vi "Hardware Out - NI 9754-1 (ESTTL).vi"(0 "FPGA Ref":T3, 11 "RT Data in":T1={"Refs"={"FPGA 1"=refnum, "FPGA 2"=refnum}, "EPT"={"MaxCAD"=0.0, "EPT Sim Enabled"=FALSE, "EPTxData"={"Sync"=FALSE, "CurrentCAD"=0.0, "Speed [RPM]"=0.0, "Config"=FALSE, "Rcvg Primary"=FALSE, "Stall"=FALSE, "Overflow"=FALSE, "Ratio Error"=FALSE, "Pattern Error"=FALSE, "Aux Warning"=FALSE, "Watchdog Error"=FALSE}}, "Raw Inputs"={"NI9752s"=[], "NI9757s"=[], "NI9411s"=[], "NI9220s"=[], "VRHalls"=[]}, "Control Inputs"={"Engine Speed [RPM]"=0.0, "Engine Status"=enum."STALLED", "Load Control \nMode"=enum."High-Idle Governor", "dt(s)"=0.0, "Number of Cylinders"=0, "Engine Displacement [cc]"=0.0, "StoichAFR"=0.0, "Q.LHV Fuel [kJ/kg]"=0.0, "BattV PSU [V]"=0.0, "12V PSU [V]"=0.0, "5V PSU [V]"=0.0, "Pedal Position [%]"=0.0, "Oil Pressure [kPa]"=0.0, "Oil Temp [C]"=0.0, "Oil Level [%]"=0.0, "Engine Coolant Temp (ECT) [C]"=0.0, "Engine Coolant Pressure [kPa]"=0.0, "Rail Pressure [bar]"=0.0, "Fuel Pressure [kPa]"=0.0, "Fuel Temp [C]"=0.0, "Vacuum Pressure [kPa]"=0.0, "Throttle Position [%]"=0.0, "Cam1 Advance [CAD]"=0.0, "Cam2 Advance [CAD]"=0.0, "Cam3 Advance [CAD]"=0.0, "Cam4 Advance [CAD]"=0.0, "CA50 Control Output [CAD]"=[], "CA50 Control Output Valid"=[], "Intake Air Temp (IAT) [C]"=0.0, "Barometric Air Pressure [kPa]"=0.0, "Intake Air Rel. Humidity [%]"=0.0, "Mass Air Flow (MAF) [kg/hr]"=0.0, "Turbo Inlet Air Pressure [kPa]"=0.0, "Turbo Inlet Air Temp [C]"=0.0, "Turbo Outlet Air Pressure [kPa]"=0.0, "Turbo Outlet Air Temp [C]"=0.0, "CAC Outlet Pressure [kPa]"=0.0, "CAC Outlet Temp [C]"=0.0, "Intake Manifold Pressure (MAP) [kPa]"=0.0, "Intake Manifold Temp (MAT) [C]"=0.0, "Exhaust Manifold Pressure [kPa]"=0.0, "Exhaust Manifold Temp [C]"=0.0, "HighP EGR Cooler Outlet Pressure [kPa]"=0.0, "HighP EGR Cooler Outlet Temp [C]"=0.0, "HighP EGR Differential Pressure [kPa]"=0.0, "HighP EGR Valve Position [%]"=0.0, "Turbo Outlet Exhaust Pressure [kPa]"=0.0, "Turbo Outlet Exhaust Temp [C]"=0.0, "VGT Position 1 [%]"=0.0, "VGT Position 2 [%]"=0.0, "Turbo Speed 1 [RPM]"=0.0, "Turbo Speed 2 [RPM]"=0.0, "LowP EGR Differential Pressure [kPa]"=0.0, "LowP EGR Valve Position [%]"=0.0, "UEGO1Lambda"=0.0, "UEGO1_Hot"=FALSE, "UEGO2Lambda"=0.0, "UEGO2_Hot"=FALSE, "Knock Intensity"=[], "Knock"=[]}, "Control Outputs"={"Pedal Desired [%]"=0.0, "MEP Desired [bar]"=0.0, "Fuel Desired [mg/cyc]"=0.0, "Intake MAP Desired [kPa]"=0.0, "Cam1 Advance Setpoint [CAD]"=0.0, "Cam2 Advance Setpoint [CAD]"=0.0, "HighP EGR Position Setpoint [%Open]"=0.0, "LowP EGR Position Setpoint [%Open]"=0.0, "Rail Pressure Setpoint [bar]"=0.0, "Wastegate1 Position Setpoint [%Open]"=0.0, "Wastegate2 Position Setpoint [%Open]"=0.0, "VGT1 Position Setpoint [%Open]"=0.0, "VGT2 Position Setpoint [%Open]"=0.0, "Throttle1 Position Setpoint [%Open]"=0.0, "Throttle2 Position Setpoint [%Open]"=0.0, "TurboBPV Position Setpoint [%Open]"=0.0, "Spark Dwells [msec]"=[], "Spark Timings [DBTDC]"=[], "PFI Quantities [mg/inj]"=[], "PFI Timings [DBTDC]"=[], "DI Quantities [mg/inj]"=[], "DI Timings [DBTDC]"=[]}, "Raw Outputs"={"9751-1"={"DI1"={"Window_Start (DBTDC)"=0.0, "Window_End (DBTDC)"=0.0, "Enable_Inj1"=FALSE, "Duration_Inj1 (msec)"=0.0, "Timing_Inj1 (DBTDC)"=0.0, "Enable_Inj2"=FALSE, "Duration_Inj2 (msec)"=0.0, "Timing_Inj2 (DBTDC)"=0.0, "Enable_Inj3"=FALSE, "Duration_Inj3 (msec)"=0.0, "Timing_Inj3 (DBTDC)"=0.0, "Enable_Inj4"=FALSE, "Duration_Inj4 (msec)"=0.0, "Timing_Inj4 (DBTDC)"=0.0, "Enable_Inj5"=FALSE, "Duration_Inj5 (msec)"=0.0, "Timing_Inj5 (DBTDC)"=0.0}, "DI2"={"Window_Start (DBTDC)"=0.0, "Window_End (DBTDC)"=0.0, "Enable_Inj1"=FALSE, "Duration_Inj1 (msec)"=0.0, "Timing_Inj1 (DBTDC)"=0.0, "Enable_Inj2"=FALSE, "Duration_Inj2 (msec)"=0.0, "Timing_Inj2 (DBTDC)"=0.0, "Enable_Inj3"=FALSE, "Duration_Inj3 (msec)"=0.0, "Timing_Inj3 (DBTDC)"=0.0, "Enable_Inj4"=FALSE, "Duration_Inj4 (msec)"=0.0, "Timing_Inj4 (DBTDC)"=0.0, "Enable_Inj5"=FALSE, "Duration_Inj5 (msec)"=0.0, "Timing_Inj5 (DBTDC)"=0.0}, "DI3"={"Window_Start (DBTDC)"=0.0, "Window_End (DBTDC)"=0.0, "Enable_Inj1"=FALSE, "Duration_Inj1 (msec)"=0.0, "Timing_Inj1 (DBTDC)"=0.0, "Enable_Inj2"=FALSE, "Duration_Inj2 (msec)"=0.0, "Timing_Inj2 (DBTDC)"=0.0, "Enable_Inj3"=FALSE, "Duration_Inj3 (msec)"=0.0, "Timing_Inj3 (DBTDC)"=0.0, "Enable_Inj4"=FALSE, "Duration_Inj4 (msec)"=0.0, "Timing_Inj4 (DBTDC)"=0.0, "Enable_Inj5"=FALSE, "Duration_Inj5 (msec)"=0.0, "Timing_Inj5 (DBTDC)"=0.0}}, "9751-2"={"DI1"={"Window_Start (DBTDC)"=0.0, "Window_End (DBTDC)"=0.0, "Enable_Inj1"=FALSE, "Duration_Inj1 (msec)"=0.0, "Timing_Inj1 (DBTDC)"=0.0, "Enable_Inj2"=FALSE, "Duration_Inj2 (msec)"=0.0, "Timing_Inj2 (DBTDC)"=0.0, "Enable_Inj3"=FALSE, "Duration_Inj3 (msec)"=0.0, "Timing_Inj3 (DBTDC)"=0.0, "Enable_Inj4"=FALSE, "Duration_Inj4 (msec)"=0.0, "Timing_Inj4 (DBTDC)"=0.0, "Enable_Inj5"=FALSE, "Duration_Inj5 (msec)"=0.0, "Timing_Inj5 (DBTDC)"=0.0}, "DI2"={"Window_Start (DBTDC)"=0.0, "Window_End (DBTDC)"=0.0, "Enable_Inj1"=FALSE, "Duration_Inj1 (msec)"=0.0, "Timing_Inj1 (DBTDC)"=0.0, "Enable_Inj2"=FALSE, "Duration_Inj2 (msec)"=0.0, "Timing_Inj2 (DBTDC)"=0.0, "Enable_Inj3"=FALSE, "Duration_Inj3 (msec)"=0.0, "Timing_Inj3 (DBTDC)"=0.0, "Enable_Inj4"=FALSE, "Duration_Inj4 (msec)"=0.0, "Timing_Inj4 (DBTDC)"=0.0, "Enable_Inj5"=FALSE, "Duration_Inj5 (msec)"=0.0, "Timing_Inj5 (DBTDC)"=0.0}, "DI3"={"Window_Start (DBTDC)"=0.0, "Window_End (DBTDC)"=0.0, "Enable_Inj1"=FALSE, "Duration_Inj1 (msec)"=0.0, "Timing_Inj1 (DBTDC)"=0.0, "Enable_Inj2"=FALSE, "Duration_Inj2 (msec)"=0.0, "Timing_Inj2 (DBTDC)"=0.0, "Enable_Inj3"=FALSE, "Duration_Inj3 (msec)"=0.0, "Timing_Inj3 (DBTDC)"=0.0, "Enable_Inj4"=FALSE, "Duration_Inj4 (msec)"=0.0, "Timing_Inj4 (DBTDC)"=0.0, "Enable_Inj5"=FALSE, "Duration_Inj5 (msec)"=0.0, "Timing_Inj5 (DBTDC)"=0.0}}, "9751-3"={"DI1"={"Window_Start (DBTDC)"=0.0, "Window_End (DBTDC)"=0.0, "Enable_Inj1"=FALSE, "Duration_Inj1 (msec)"=0.0, "Timing_Inj1 (DBTDC)"=0.0, "Enable_Inj2"=FALSE, "Duration_Inj2 (msec)"=0.0, "Timing_Inj2 (DBTDC)"=0.0, "Enable_Inj3"=FALSE, "Duration_Inj3 (msec)"=0.0, "Timing_Inj3 (DBTDC)"=0.0, "Enable_Inj4"=FALSE, "Duration_Inj4 (msec)"=0.0, "Timing_Inj4 (DBTDC)"=0.0, "Enable_Inj5"=FALSE, "Duration_Inj5 (msec)"=0.0, "Timing_Inj5 (DBTDC)"=0.0}, "DI2"={"Window_Start (DBTDC)"=0.0, "Window_End (DBTDC)"=0.0, "Enable_Inj1"=FALSE, "Duration_Inj1 (msec)"=0.0, "Timing_Inj1 (DBTDC)"=0.0, "Enable_Inj2"=FALSE, "Duration_Inj2 (msec)"=0.0, "Timing_Inj2 (DBTDC)"=0.0, "Enable_Inj3"=FALSE, "Duration_Inj3 (msec)"=0.0, "Timing_Inj3 (DBTDC)"=0.0, "Enable_Inj4"=FALSE, "Duration_Inj4 (msec)"=0.0, "Timing_Inj4 (DBTDC)"=0.0, "Enable_Inj5"=FALSE, "Duration_Inj5 (msec)"=0.0, "Timing_Inj5 (DBTDC)"=0.0}, "DI3"={"Window_Start (DBTDC)"=0.0, "Window_End (DBTDC)"=0.0, "Enable_Inj1"=FALSE, "Duration_Inj1 (msec)"=0.0, "Timing_Inj1 (DBTDC)"=0.0, "Enable_Inj2"=FALSE, "Duration_Inj2 (msec)"=0.0, "Timing_Inj2 (DBTDC)"=0.0, "Enable_Inj3"=FALSE, "Duration_Inj3 (msec)"=0.0, "Timing_Inj3 (DBTDC)"=0.0, "Enable_Inj4"=FALSE, "Duration_Inj4 (msec)"=0.0, "Timing_Inj4 (DBTDC)"=0.0, "Enable_Inj5"=FALSE, "Duration_Inj5 (msec)"=0.0, "Timing_Inj5 (DBTDC)"=0.0}}, "9751-4"={"DI1"={"Window_Start (DBTDC)"=0.0, "Window_End (DBTDC)"=0.0, "Enable_Inj1"=FALSE, "Duration_Inj1 (msec)"=0.0, "Timing_Inj1 (DBTDC)"=0.0, "Enable_Inj2"=FALSE, "Duration_Inj2 (msec)"=0.0, "Timing_Inj2 (DBTDC)"=0.0, "Enable_Inj3"=FALSE, "Duration_Inj3 (msec)"=0.0, "Timing_Inj3 (DBTDC)"=0.0, "Enable_Inj4"=FALSE, "Duration_Inj4 (msec)"=0.0, "Timing_Inj4 (DBTDC)"=0.0, "Enable_Inj5"=FALSE, "Duration_Inj5 (msec)"=0.0, "Timing_Inj5 (DBTDC)"=0.0}, "DI2"={"Window_Start (DBTDC)"=0.0, "Window_End (DBTDC)"=0.0, "Enable_Inj1"=FALSE, "Duration_Inj1 (msec)"=0.0, "Timing_Inj1 (DBTDC)"=0.0, "Enable_Inj2"=FALSE, "Duration_Inj2 (msec)"=0.0, "Timing_Inj2 (DBTDC)"=0.0, "Enable_Inj3"=FALSE, "Duration_Inj3 (msec)"=0.0, "Timing_Inj3 (DBTDC)"=0.0, "Enable_Inj4"=FALSE, "Duration_Inj4 (msec)"=0.0, "Timing_Inj4 (DBTDC)"=0.0, "Enable_Inj5"=FALSE, "Duration_Inj5 (msec)"=0.0, "Timing_Inj5 (DBTDC)"=0.0}, "DI3"={"Window_Start (DBTDC)"=0.0, "Window_End (DBTDC)"=0.0, "Enable_Inj1"=FALSE, "Duration_Inj1 (msec)"=0.0, "Timing_Inj1 (DBTDC)"=0.0, "Enable_Inj2"=FALSE, "Duration_Inj2 (msec)"=0.0, "Timing_Inj2 (DBTDC)"=0.0, "Enable_Inj3"=FALSE, "Duration_Inj3 (msec)"=0.0, "Timing_Inj3 (DBTDC)"=0.0, "Enable_Inj4"=FALSE, "Duration_Inj4 (msec)"=0.0, "Timing_Inj4 (DBTDC)"=0.0, "Enable_Inj5"=FALSE, "Duration_Inj5 (msec)"=0.0, "Timing_Inj5 (DBTDC)"=0.0}}, "9754-1"={"ESTTL 1"={"Timing (DBTDC)"=0.0, "Dwell (ms)"=0.0}, "ESTTL 2"={"Timing (DBTDC)"=0.0, "Dwell (ms)"=0.0}, "ESTTL 3"={"Timing (DBTDC)"=0.0, "Dwell (ms)"=0.0}, "ESTTL 4"={"Timing (DBTDC)"=0.0, "Dwell (ms)"=0.0}, "ESTTL 5"={"Timing (DBTDC)"=0.0, "Dwell (ms)"=0.0}, "ESTTL 6"={"Timing (DBTDC)"=0.0, "Dwell (ms)"=0.0}, "ESTTL 7"={"Timing (DBTDC)"=0.0, "Dwell (ms)"=0.0}, "ESTTL 8"={"Timing (DBTDC)"=0.0, "Dwell (ms)"=0.0}}, "9754-2"={"ESTTL 1"={"Timing (DBTDC)"=0.0, "Dwell (ms)"=0.0}, "ESTTL 2"={"Timing (DBTDC)"=0.0, "Dwell (ms)"=0.0}, "ESTTL 3"={"Timing (DBTDC)"=0.0, "Dwell (ms)"=0.0}, "ESTTL 4"={"Timing (DBTDC)"=0.0, "Dwell (ms)"=0.0}, "ESTTL 5"={"Timing (DBTDC)"=0.0, "Dwell (ms)"=0.0}, "ESTTL 6"={"Timing (DBTDC)"=0.0, "Dwell (ms)"=0.0}, "ESTTL 7"={"Timing (DBTDC)"=0.0, "Dwell (ms)"=0.0}, "ESTTL 8"={"Timing (DBTDC)"=0.0, "Dwell (ms)"=0.0}}, "9758-1"={"LS 1"={"Enable"=FALSE, "Freq [Hz]"=0.0, "DutyCyc [%]"=0.0}, "LS 2"={"Enable"=FALSE, "Freq [Hz]"=0.0, "DutyCyc [%]"=0.0}, "LS 3"={"Enable"=FALSE, "Freq [Hz]"=0.0, "DutyCyc [%]"=0.0}, "LS 4"={"Enable"=FALSE, "Freq [Hz]"=0.0, "DutyCyc [%]"=0.0}, "PFI 1"={"Position Mode"=FALSE, "Timing (DBTDC)"=0.0, "Pulse Width (ms)"=0.0}, "PFI 2"={"Position Mode"=FALSE, "Timing (DBTDC)"=0.0, "Pulse Width (ms)"=0.0}, "PFI 3"={"Position Mode"=FALSE, "Timing (DBTDC)"=0.0, "Pulse Width (ms)"=0.0}, "PFI 4"={"Position Mode"=FALSE, "Timing (DBTDC)"=0.0, "Pulse Width (ms)"=0.0}}, "9758-2"={"LS 1"={"Enable"=FALSE, "Freq [Hz]"=0.0, "DutyCyc [%]"=0.0}, "LS 2"={"Enable"=FALSE, "Freq [Hz]"=0.0, "DutyCyc [%]"=0.0}, "LS 3"={"Enable"=FALSE, "Freq [Hz]"=0.0, "DutyCyc [%]"=0.0}, "LS 4"={"Enable"=FALSE, "Freq [Hz]"=0.0, "DutyCyc [%]"=0.0}, "PFI 1"={"Position Mode"=FALSE, "Timing (DBTDC)"=0.0, "Pulse Width (ms)"=0.0}, "PFI 2"={"Position Mode"=FALSE, "Timing (DBTDC)"=0.0, "Pulse Width (ms)"=0.0}, "PFI 3"={"Position Mode"=FALSE, "Timing (DBTDC)"=0.0, "Pulse Width (ms)"=0.0}, "PFI 4"={"Position Mode"=FALSE, "Timing (DBTDC)"=0.0, "Pulse Width (ms)"=0.0}}, "9759-1"={"THR1-1 DC [%]"=0.0, "THR1-1 Setpoint [% Open]"=0.0, "THR1-2 DC [%]"=0.0, "THR1-2 Setpoint [% Open]"=0.0}}} {"Control Inputs"."Knock Intensity" format="%.2f"; "Control Inputs"."CA50 Control Output [CAD]" format="%.2f"; "Control Inputs"."Exhaust Manifold Temp [C]" format="%#_6f"; "Control Inputs"."UEGO2Lambda" format="%.2f"; "Control Inputs"."Intake Manifold Temp (MAT) [C]" format="%#_6f"; "Control Inputs"."UEGO1Lambda" format="%.2f"}) -> ()   [LabVIEW 2015, in "ECS-RT.lvlib"]
uses:
  ECS-RT.lvlib
  Typedefs/FPGA Refs/Generic FPGA Ref.ctl
  Typedefs/RT Data.ctl
  Typedefs/FPGA Refs/FPGA Refs.ctl
  Typedefs/EPT/EPT Cluster.ctl
  <vilib>/Powertrain Controls/Device Drivers/Engine Position Tracking/EPTx/RevA/RT/Controls/EPTxData.ctl
  Typedefs/Raw Inputs/Raw Inputs.ctl
  Typedefs/Raw Inputs/NI9752.ctl
  Typedefs/Raw Inputs/PPWData.ctl
  Typedefs/Raw Inputs/NI9757.ctl
  Typedefs/Raw Inputs/NI9411.ctl
  Typedefs/Raw Inputs/NI9220.ctl
  Typedefs/Raw Inputs/VRHall.ctl
  Typedefs/Control Inputs/Control Inputs.ctl
  Typedefs/EPT/Engine Status.ctl
  Typedefs/MISC/Load Control Mode.ctl
  Typedefs/Control Outputs/Control Outputs.ctl
  Typedefs/Control Outputs/Injection Quantity.ctl
  Typedefs/Control Outputs/Injection Timing.ctl
  Typedefs/Raw Outputs/Raw Outputs.ctl
  Typedefs/Raw Outputs/NI9751.ctl
  Typedefs/Raw Outputs/DI.ctl
  Typedefs/Raw Outputs/NI9754.ctl
  Typedefs/Raw Outputs/ESTTL.ctl
  Typedefs/Raw Outputs/NI9758.ctl
  Typedefs/Raw Outputs/LS.ctl
  Typedefs/Raw Outputs/PFI.ctl
  Typedefs/Raw Outputs/NI9759.ctl
  <vilib>/Utility/error.llb/Error Cluster From Error Code.vi
  <vilib>/rvi/errors/niLvFpgaAdjustHostInterfaceError.vi
  Globals/TDC Globals.vi
  <vilib>/rvi/interface/nirviReadWriteControl/nirviReadWriteControl.xnode
  <vilib>/rvi/interface/Simulation/niFpgaSimulationCallBeginRW.vi
  NiFpgaLv.dll
  <vilib>/Powertrain Controls/Device Drivers/Engine Position Tracking/EPTx/RevA/RT/EPTx - RevA - RT.lvlib
  ECS-Shared.lvlib
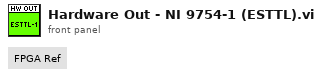
[diagram p1: front panel]
types:
  T1 = typedef "ECS-Shared.lvlib/RT Data.ctl" = cluster{"Refs":T2, "EPT":T4, "Raw Inputs":T6, "Control Inputs":T13, "Control Outputs":T16, "Raw Outputs":T19}
  T2 = typedef "ECS-Shared.lvlib/FPGA Refs.ctl" = cluster{"FPGA 1":T3, "FPGA 2":T3}
  T3 = typedef "ECS-Shared.lvlib/Generic FPGA Ref.ctl" = refnum<k20>
  T4 = typedef "ECS-Shared.lvlib/EPT Cluster.ctl" = cluster{"MaxCAD":sgl, "EPT Sim Enabled":bool, "EPTxData":T5}
  T5 = typedef "EPTx - RevA - RT.lvlib/EPTxData.ctl" = cluster{"Sync":bool, "CurrentCAD":sgl, "Speed [RPM]":sgl, "Config":bool, "Rcvg Primary":bool, "Stall":bool, "Overflow":bool, "Ratio Error":bool, "Pattern Error":bool, "Aux Warning":bool, "Watchdog Error":bool}
  T6 = typedef "ECS-Shared.lvlib/Raw Inputs.ctl" = cluster{"NI9752s":T7[], "NI9757s":T9[], "NI9411s":T10[], "NI9220s":T11[], "VRHalls":T12[]}
  T7 = typedef "ECS-Shared.lvlib/NI9752.ctl" = cluster{"Voltage [V]":sgl[], "Resistance [Ohm]":sgl[], "PPWData VR1":T8, "PPWData VR2":T8, "PPWData Hall1":T8, "PPWData Hall2":T8}
  T8 = typedef "ECS-Shared.lvlib/PPWData.ctl" = cluster{"Period":u32, "PulseWidth":u32, "Stopped":bool}
  T9 = typedef "ECS-Shared.lvlib/NI9757.ctl" = cluster{"UEGO1":cluster{"Lambda":sgl, "Phi":sgl, "AF_Ratio":sgl, "Ip":sgl, "Temp":sgl, "Hot":bool}, "UEGO2":cluster{"Lambda":sgl, "Phi":sgl, "AF_Ratio":sgl, "Ip":sgl, "Temp":sgl, "Hot":bool}, "EGO1":cluster{"Status":enum16{"COLD SENSOR", "FOULED SENSOR", "RICH", "LEAN"}, "SensorV":sgl}, "EGO2":cluster{"Status":enum16{"COLD SENSOR", "FOULED SENSOR", "RICH", "LEAN"}, "SensorV":sgl}, "EGO3":cluster{"Status":enum16{"COLD SENSOR", "FOULED SENSOR", "RICH", "LEAN"}, "SensorV":sgl}, "EGO4":cluster{"Status":enum16{"COLD SENSOR", "FOULED SENSOR", "RICH", "LEAN"}, "SensorV":sgl}}
  T10 = typedef "ECS-Shared.lvlib/NI9411.ctl" = cluster{"PPWData 0":T8, "PPWData 1":T8, "PPWData 2":T8, "PPWData 3":T8, "PPWData 4":T8, "PPWData 5":T8}
  T11 = typedef "ECS-Shared.lvlib/NI9220.ctl" = cluster{"AI 0":sgl, "AI 1":sgl, "AI 2":sgl, "AI 3":sgl, "AI 4":sgl, "AI 5":sgl, "AI 6":sgl, "AI 7":sgl, "AI 8":sgl, "AI 9":sgl, "AI 10":sgl, "AI 11":sgl, "AI 12":sgl, "AI 13":sgl, "AI 14":sgl, "AI 15":sgl}
  T12 = typedef "ECS-Shared.lvlib/VRHall.ctl" = cluster{"PPWData 0":T8, "PPWData 1":T8, "PPWData 2":T8, "PPWData 3":T8, "PPWData 4":T8, "PPWData 5":T8}
  T13 = typedef "ECS-Shared.lvlib/Control Inputs.ctl" = cluster{"Engine Speed [RPM]":sgl, "Engine Status":T14, "Load Control \nMode":T15, "dt(s)":sgl, "Number of Cylinders":u8, "Engine Displacement [cc]":sgl, "StoichAFR":sgl, "Q.LHV Fuel [kJ/kg]":sgl, "BattV PSU [V]":sgl, "12V PSU [V]":sgl, "5V PSU [V]":sgl, "Pedal Position [%]":sgl, "Oil Pressure [kPa]":sgl, "Oil Temp [C]":sgl, "Oil Level [%]":sgl, "Engine Coolant Temp (ECT) [C]":sgl, "Engine Coolant Pressure [kPa]":sgl, "Rail Pressure [bar]":sgl, "Fuel Pressure [kPa]":sgl, "Fuel Temp [C]":sgl, "Vacuum Pressure [kPa]":sgl, "Throttle Position [%]":sgl, "Cam1 Advance [CAD]":sgl, "Cam2 Advance [CAD]":sgl, "Cam3 Advance [CAD]":sgl, "Cam4 Advance [CAD]":sgl, "CA50 Control Output [CAD]":sgl[], "CA50 Control Output Valid":bool[], "Intake Air Temp (IAT) [C]":sgl, "Barometric Air Pressure [kPa]":sgl, "Intake Air Rel. Humidity [%]":sgl, "Mass Air Flow (MAF) [kg/hr]":sgl, "Turbo Inlet Air Pressure [kPa]":sgl, "Turbo Inlet Air Temp [C]":sgl, "Turbo Outlet Air Pressure [kPa]":sgl, "Turbo Outlet Air Temp [C]":sgl, "CAC Outlet Pressure [kPa]":sgl, "CAC Outlet Temp [C]":sgl, "Intake Manifold Pressure (MAP) [kPa]":sgl, "Intake Manifold Temp (MAT) [C]":sgl, "Exhaust Manifold Pressure [kPa]":sgl, "Exhaust Manifold Temp [C]":sgl, "HighP EGR Cooler Outlet Pressure [kPa]":sgl, "HighP EGR Cooler Outlet Temp [C]":sgl, "HighP EGR Differential Pressure [kPa]":sgl, "HighP EGR Valve Position [%]":sgl, "Turbo Outlet Exhaust Pressure [kPa]":sgl, "Turbo Outlet Exhaust Temp [C]":sgl, "VGT Position 1 [%]":sgl, "VGT Position 2 [%]":sgl, "Turbo Speed 1 [RPM]":sgl, "Turbo Speed 2 [RPM]":sgl, "LowP EGR Differential Pressure [kPa]":sgl, "LowP EGR Valve Position [%]":sgl, "UEGO1Lambda":sgl, "UEGO1_Hot":bool, "UEGO2Lambda":sgl, "UEGO2_Hot":bool, "Knock Intensity":sgl[], "Knock":bool[]}
  T14 = typedef "ECS-Shared.lvlib/Engine Status.ctl" = enum16{"OFF", "STALLED", "CRANKING", "RUNNING", "ACCEL", "DECEL", "SAFE"}
  T15 = typedef "ECS-Shared.lvlib/Load Control Mode.ctl" = enum16{"No Governor", "Low-Idle Governor", "High-Idle Governor"}
  T16 = typedef "ECS-Shared.lvlib/Control Outputs.ctl" = cluster{"Pedal Desired [%]":sgl, "MEP Desired [bar]":sgl, "Fuel Desired [mg/cyc]":sgl, "Intake MAP Desired [kPa]":sgl, "Cam1 Advance Setpoint [CAD]":sgl, "Cam2 Advance Setpoint [CAD]":sgl, "HighP EGR Position Setpoint [%Open]":sgl, "LowP EGR Position Setpoint [%Open]":sgl, "Rail Pressure Setpoint [bar]":sgl, "Wastegate1 Position Setpoint [%Open]":sgl, "Wastegate2 Position Setpoint [%Open]":sgl, "VGT1 Position Setpoint [%Open]":sgl, "VGT2 Position Setpoint [%Open]":sgl, "Throttle1 Position Setpoint [%Open]":sgl, "Throttle2 Position Setpoint [%Open]":sgl, "TurboBPV Position Setpoint [%Open]":sgl, "Spark Dwells [msec]":sgl[], "Spark Timings [DBTDC]":sgl[], "PFI Quantities [mg/inj]":sgl[], "PFI Timings [DBTDC]":sgl[], "DI Quantities [mg/inj]":T17[], "DI Timings [DBTDC]":T18[]}
  T17 = typedef "ECS-Shared.lvlib/Injection Quantity.ctl" = cluster{"Pilot1Quantity [mg/inj]":sgl, "Pilot2Quantity [mg/inj]":sgl, "MainQuantity [mg/inj]":sgl, "Post1Quantity [mg/inj]":sgl, "Post2Quantity [mg/inj]":sgl}
  T18 = typedef "ECS-Shared.lvlib/Injection Timing.ctl" = cluster{"Pilot1SOI [DBTDC]":sgl, "Pilot2SOI [DBTDC]":sgl, "MainSOI [DBTDC]":sgl, "Post1SOI [DBTDC]":sgl, "Post2SOI [DBTDC]":sgl}
  T19 = typedef "ECS-Shared.lvlib/Raw Outputs.ctl" = cluster{"9751-1":T20, "9751-2":T20, "9751-3":T20, "9751-4":T20, "9754-1":T22, "9754-2":T22, "9758-1":T24, "9758-2":T24, "9759-1":T27}
  T20 = typedef "ECS-Shared.lvlib/NI9751.ctl" = cluster{"DI1":T21, "DI2":T21, "DI3":T21}
  T21 = typedef "ECS-Shared.lvlib/DI.ctl" = cluster{"Window_Start (DBTDC)":sgl, "Window_End (DBTDC)":sgl, "Enable_Inj1":bool, "Duration_Inj1 (msec)":sgl, "Timing_Inj1 (DBTDC)":sgl, "Enable_Inj2":bool, "Duration_Inj2 (msec)":sgl, "Timing_Inj2 (DBTDC)":sgl, "Enable_Inj3":bool, "Duration_Inj3 (msec)":sgl, "Timing_Inj3 (DBTDC)":sgl, "Enable_Inj4":bool, "Duration_Inj4 (msec)":sgl, "Timing_Inj4 (DBTDC)":sgl, "Enable_Inj5":bool, "Duration_Inj5 (msec)":sgl, "Timing_Inj5 (DBTDC)":sgl}
  T22 = typedef "ECS-Shared.lvlib/NI9754.ctl" = cluster{"ESTTL 1":T23, "ESTTL 2":T23, "ESTTL 3":T23, "ESTTL 4":T23, "ESTTL 5":T23, "ESTTL 6":T23, "ESTTL 7":T23, "ESTTL 8":T23}
  T23 = typedef "ECS-Shared.lvlib/ESTTL.ctl" = cluster{"Timing (DBTDC)":sgl, "Dwell (ms)":sgl}
  T24 = typedef "ECS-Shared.lvlib/NI9758.ctl" = cluster{"LS 1":T25, "LS 2":T25, "LS 3":T25, "LS 4":T25, "PFI 1":T26, "PFI 2":T26, "PFI 3":T26, "PFI 4":T26}
  T25 = typedef "ECS-Shared.lvlib/LS.ctl" = cluster{"Enable":bool, "Freq [Hz]":sgl, "DutyCyc [%]":sgl}
  T26 = typedef "ECS-Shared.lvlib/PFI.ctl" = cluster{"Position Mode":bool, "Timing (DBTDC)":sgl, "Pulse Width (ms)":sgl}
  T27 = typedef "ECS-Shared.lvlib/NI9759.ctl" = cluster{"THR1-1 DC [%]":sgl, "THR1-1 Setpoint [% Open]":sgl, "THR1-2 DC [%]":sgl, "THR1-2 Setpoint [% Open]":sgl}
  T28 = cluster{"Channel Enable 1":bool, "Window_Start 1 [CAD]":fxp<+,18,11>, "Window_End 1 [CAD]":fxp<+,18,11>, "Dwell 1 [ms]":fxp<+/-,22,9>, "Spark Timing 1 [CAD]":fxp<+,18,11>, "Channel Enable 2":bool, "Window_Start 2 [CAD]":fxp<+,18,11>, "Window_End 2 [CAD]":fxp<+,18,11>, "Dwell 2 [ms]":fxp<+/-,22,9>, "Spark Timing 2 [CAD]":fxp<+,18,11>, "Channel Enable 3":bool, "Window_Start 3 [CAD]":fxp<+,18,11>, "Window_End 3 [CAD]":fxp<+,18,11>, "Dwell 3 [ms]":fxp<+/-,22,9>, "Spark Timing 3 [CAD]":fxp<+,18,11>, "Channel Enable 4":bool, "Window_Start 4 [CAD]":fxp<+,18,11>, "Window_End 4 [CAD]":fxp<+,18,11>, "Dwell 4 [ms]":fxp<+/-,22,9>, "Spark Timing 4 [CAD]":fxp<+,18,11>, "Channel Enable 5":bool, "Window_Start 5 [CAD]":fxp<+,18,11>, "Window_End 5 [CAD]":fxp<+,18,11>, "Dwell 5 [ms]":fxp<+/-,22,9>, "Spark Timing 5 [CAD]":fxp<+,18,11>, "Channel Enable 6":bool, "Window_Start 6 [CAD]":fxp<+,18,11>, "Window_End 6 [CAD]":fxp<+,18,11>, "Dwell 6 [ms]":fxp<+/-,22,9>, "Spark Timing 6 [CAD]":fxp<+,18,11>, "Channel Enable 7":bool, "Window_Start 7 [CAD]":fxp<+,18,11>, "Window_End 7 [CAD]":fxp<+,18,11>, "Dwell 7 [ms]":fxp<+/-,22,9>, "Spark Timing 7 [CAD]":fxp<+,18,11>, "Channel Enable 8":bool, "Window_Start 8 [CAD]":fxp<+,18,11>, "Window_End 8 [CAD]":fxp<+,18,11>, "Dwell 8 [ms]":fxp<+/-,22,9>, "Spark Timing 8 [CAD]":fxp<+,18,11>}
  T29 = cluster{"DurationSeq":u32[], "CmdLevelSeq":bool[], "ContinueSeq":bool[]}
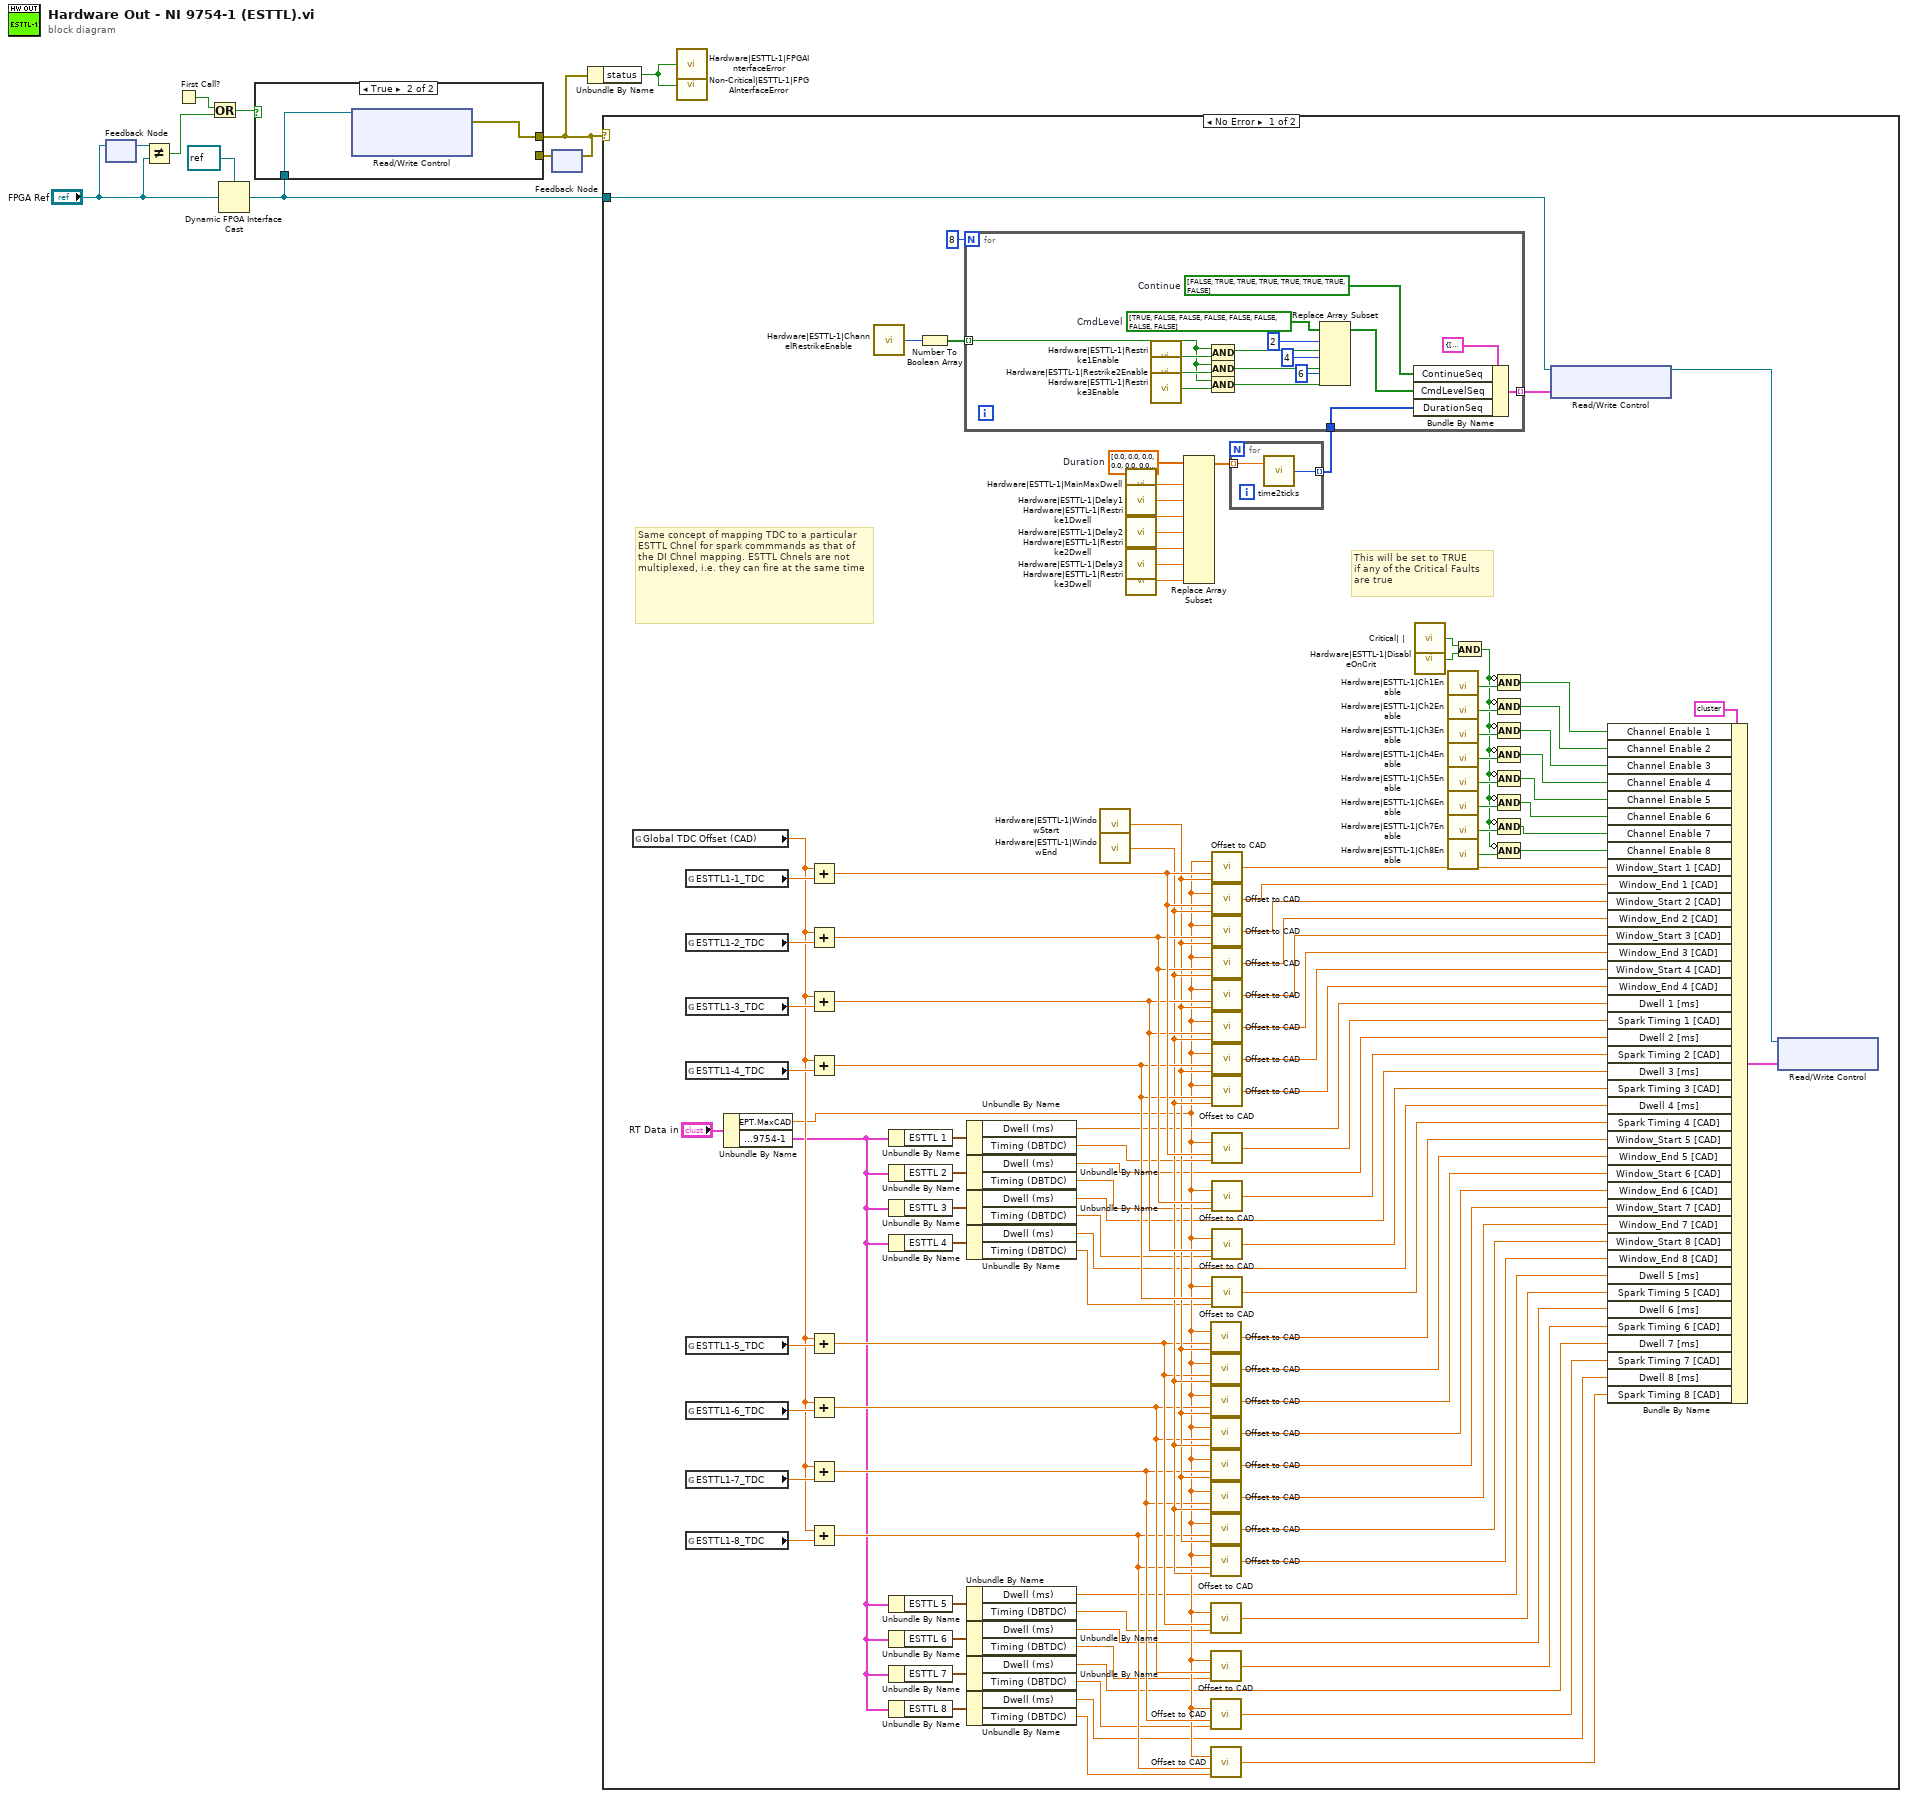
[diagram p0: block diagram]
diagram:
  n1 = feedback #1() -> (w7:T3)  [unwired: 1 in]
  n2 = feedback-in #1("FPGA Ref") -> ()
  n3 = Not Equal?(x=w7, y="FPGA Ref") -> (x != y?=w6:bool)
  n4 = First Call?() -> (First Call?: T/F=w8:bool)
  n5 = Or(x=w8, y=w6) -> (x .or. y?=w9:bool)
  n6 = Dynamic FPGA Interface Cast(Session In=refnum<k20> refnum ("NI 9754 (ESTTL)"), Type="FPGA Ref") -> (Session Out=w5:refnum<k20>)
  n7 = feedback #2() -> (w10:errorcluster)  [unwired: 1 in]
  n8 = case shown="True" w9 {
    tunnel: [w11 w13] -> w2
    tunnel: w10 -> [w11 _]
    tunnel: w5 -> [_ w12]
    frame False {
    }
    frame True {
      n9 = xnode "Read/Write Control"("FPGA VI Reference In"=w12) -> ("error out"=w13:errorcluster)  [unwired: 3 in, 1 out]
    }
  }
  n10 = feedback-in #2(w2) -> ()
  n11 = Unbundle By Name(w2) -> ("status"=w1:bool)
  n12 = case shown="No Error" w2 {
    tunnel: w5 -> [w65 _]
    frame No Error {
      w53 = sgl[] [0.0, 0.0, 0.0, 0.0, 0.0, 0.0, 0.0, 0.0]  # Duration
      # "This will be set to TRUE\nif any of the Critical Faults\nare true"
      # "Same concept of mapping TDC to a particular ESTTL Chnel for spark commmands as that of the DI Chnel mapping. ESTTL Chnels are not multiplexed, i.e. they can fire at the same time"
      n13 = global read "TDC Globals.vi" "Global TDC Offset (CAD)"() -> (w66:sgl)
      n14 = global read "TDC Globals.vi" "ESTTL1-1_TDC"() -> (w78:sgl)
      n15 = global read "TDC Globals.vi" "ESTTL1-2_TDC"() -> (w77:sgl)
      n16 = global read "TDC Globals.vi" "ESTTL1-3_TDC"() -> (w76:sgl)
      n17 = global read "TDC Globals.vi" "ESTTL1-4_TDC"() -> (w75:sgl)
      n18 = global read "TDC Globals.vi" "ESTTL1-5_TDC"() -> (w74:sgl)
      n19 = global read "TDC Globals.vi" "ESTTL1-6_TDC"() -> (w73:sgl)
      n20 = global read "TDC Globals.vi" "ESTTL1-7_TDC"() -> (w72:sgl)
      n21 = global read "TDC Globals.vi" "ESTTL1-8_TDC"() -> (w71:sgl)
      n22 = Unbundle By Name("RT Data in") -> ("EPT.MaxCAD"=w42:sgl, "Raw Outputs.9754-1"=w19:T22)
      n23 = Add(x=w66, y=w78) -> (x+y=w104:sgl)
      n24 = Add(x=w66, y=w77) -> (x+y=w103:sgl)
      n25 = Add(x=w66, y=w76) -> (x+y=w102:sgl)
      n26 = Add(x=w66, y=w75) -> (x+y=w101:sgl)
      n27 = Add(x=w66, y=w74) -> (x+y=w94:sgl)
      n28 = Add(x=w66, y=w73) -> (x+y=w93:sgl)
      n29 = Add(x=w66, y=w72) -> (x+y=w92:sgl)
      n30 = Add(x=w66, y=w71) -> (x+y=w91:sgl)
      n31 = call "Hardware|ESTTL-1|ChannelRestrikeEnable"() -> ("Value"=w68:u8)
      n32 = Unbundle By Name(w19) -> ("ESTTL 1"=w35:T23)
      n33 = Unbundle By Name(w19) -> ("ESTTL 2"=w34:T23)
      n34 = Unbundle By Name(w19) -> ("ESTTL 3"=w33:T23)
      n35 = Unbundle By Name(w19) -> ("ESTTL 4"=w32:T23)
      n36 = Unbundle By Name(w19) -> ("ESTTL 5"=w28:T23)
      n37 = Unbundle By Name(w19) -> ("ESTTL 6"=w29:T23)
      n38 = Unbundle By Name(w19) -> ("ESTTL 7"=w30:T23)
      n39 = Unbundle By Name(w19) -> ("ESTTL 8"=w31:T23)
      n40 = Number To Boolean Array(number=w68) -> (Boolean array=w69:bool[])
      n41 = Unbundle By Name(w35) -> ("Dwell (ms)"=w63:sgl, "Timing (DBTDC)"=w70:sgl)
      n42 = Unbundle By Name(w34) -> ("Dwell (ms)"=w41:sgl, "Timing (DBTDC)"=w40:sgl)
      n43 = Unbundle By Name(w33) -> ("Dwell (ms)"=w39:sgl, "Timing (DBTDC)"=w38:sgl)
      n44 = Unbundle By Name(w32) -> ("Dwell (ms)"=w37:sgl, "Timing (DBTDC)"=w36:sgl)
      n45 = Unbundle By Name(w28) -> ("Dwell (ms)"=w27:sgl, "Timing (DBTDC)"=w25:sgl)
      n46 = Unbundle By Name(w29) -> ("Dwell (ms)"=w26:sgl, "Timing (DBTDC)"=w24:sgl)
      n47 = Unbundle By Name(w30) -> ("Dwell (ms)"=w23:sgl, "Timing (DBTDC)"=w22:sgl)
      n48 = Unbundle By Name(w31) -> ("Dwell (ms)"=w21:sgl, "Timing (DBTDC)"=w20:sgl)
      n49 = call "Hardware|ESTTL-1|WindowStart"() -> ("Value"=w95:sgl)
      n50 = call "Hardware|ESTTL-1|WindowEnd"() -> ("Value"=w96:sgl)
      n51 = call "Hardware|ESTTL-1|MainMaxDwell"() -> ("Value"=w46:sgl)
      n52 = call "Hardware|ESTTL-1|Delay1"() -> ("Value"=w47:sgl)
      n53 = call "Hardware|ESTTL-1|Restrike1Dwell"() -> ("Value"=w48:sgl)
      n54 = call "Hardware|ESTTL-1|Delay2"() -> ("Value"=w49:sgl)
      n55 = call "Hardware|ESTTL-1|Restrike2Dwell"() -> ("Value"=w50:sgl)
      n56 = call "Hardware|ESTTL-1|Delay3"() -> ("Value"=w51:sgl)
      n57 = call "Hardware|ESTTL-1|Restrike3Dwell"() -> ("Value"=w52:sgl)
      n58 = Replace Array Subset(array=w53, new element #1=w46, new element #2=w47, new element #3=w48, new element #4=w49, new element #5=w50, new element #6=w51, new element #7=w52) -> (w45:sgl[])  [unwired: 7 in]
      n59 = call <vilib>:"Offset to CAD.vi"("Max CAD"=w42, "Cylinder TDC [Absolute CAD]"=w94, "Offset [DBTDC]"=w95) -> ("CAD [Absolute CAD]"=w90:sgl)  [unwired: 12 in]
      n60 = call <vilib>:"Offset to CAD.vi"("Max CAD"=w42, "Cylinder TDC [Absolute CAD]"=w94, "Offset [DBTDC]"=w96) -> ("CAD [Absolute CAD]"=w89:sgl)  [unwired: 12 in]
      n61 = call <vilib>:"Offset to CAD.vi"("Max CAD"=w42, "Cylinder TDC [Absolute CAD]"=w93, "Offset [DBTDC]"=w95) -> ("CAD [Absolute CAD]"=w88:sgl)  [unwired: 12 in]
      n62 = call <vilib>:"Offset to CAD.vi"("Max CAD"=w42, "Cylinder TDC [Absolute CAD]"=w93, "Offset [DBTDC]"=w96) -> ("CAD [Absolute CAD]"=w87:sgl)  [unwired: 12 in]
      n63 = call <vilib>:"Offset to CAD.vi"("Max CAD"=w42, "Cylinder TDC [Absolute CAD]"=w92, "Offset [DBTDC]"=w95) -> ("CAD [Absolute CAD]"=w86:sgl)  [unwired: 12 in]
      n64 = call <vilib>:"Offset to CAD.vi"("Max CAD"=w42, "Cylinder TDC [Absolute CAD]"=w92, "Offset [DBTDC]"=w96) -> ("CAD [Absolute CAD]"=w85:sgl)  [unwired: 12 in]
      n65 = call <vilib>:"Offset to CAD.vi"("Max CAD"=w42, "Cylinder TDC [Absolute CAD]"=w91, "Offset [DBTDC]"=w95) -> ("CAD [Absolute CAD]"=w84:sgl)  [unwired: 12 in]
      n66 = call <vilib>:"Offset to CAD.vi"("Max CAD"=w42, "Cylinder TDC [Absolute CAD]"=w91, "Offset [DBTDC]"=w96) -> ("CAD [Absolute CAD]"=w83:sgl)  [unwired: 12 in]
      n67 = call <vilib>:"Offset to CAD.vi"("Max CAD"=w42, "Cylinder TDC [Absolute CAD]"=w94, "Offset [DBTDC]"=w25) -> ("CAD [Absolute CAD]"=w82:sgl)  [unwired: 12 in]
      n68 = call <vilib>:"Offset to CAD.vi"("Max CAD"=w42, "Cylinder TDC [Absolute CAD]"=w93, "Offset [DBTDC]"=w24) -> ("CAD [Absolute CAD]"=w81:sgl)  [unwired: 12 in]
      n69 = call <vilib>:"Offset to CAD.vi"("Max CAD"=w42, "Cylinder TDC [Absolute CAD]"=w92, "Offset [DBTDC]"=w22) -> ("CAD [Absolute CAD]"=w80:sgl)  [unwired: 12 in]
      n70 = call <vilib>:"Offset to CAD.vi"("Max CAD"=w42, "Cylinder TDC [Absolute CAD]"=w91, "Offset [DBTDC]"=w20) -> ("CAD [Absolute CAD]"=w79:sgl)  [unwired: 12 in]
      n71 = call <vilib>:"Offset to CAD.vi"("Max CAD"=w42, "Cylinder TDC [Absolute CAD]"=w104, "Offset [DBTDC]"=w95) -> ("CAD [Absolute CAD]"=w119:sgl)  [unwired: 12 in]
      n72 = call <vilib>:"Offset to CAD.vi"("Max CAD"=w42, "Cylinder TDC [Absolute CAD]"=w104, "Offset [DBTDC]"=w96) -> ("CAD [Absolute CAD]"=w118:sgl)  [unwired: 12 in]
      n73 = call <vilib>:"Offset to CAD.vi"("Max CAD"=w42, "Cylinder TDC [Absolute CAD]"=w103, "Offset [DBTDC]"=w95) -> ("CAD [Absolute CAD]"=w117:sgl)  [unwired: 12 in]
      n74 = call <vilib>:"Offset to CAD.vi"("Max CAD"=w42, "Cylinder TDC [Absolute CAD]"=w103, "Offset [DBTDC]"=w96) -> ("CAD [Absolute CAD]"=w116:sgl)  [unwired: 12 in]
      n75 = call <vilib>:"Offset to CAD.vi"("Max CAD"=w42, "Cylinder TDC [Absolute CAD]"=w102, "Offset [DBTDC]"=w95) -> ("CAD [Absolute CAD]"=w115:sgl)  [unwired: 12 in]
      n76 = call <vilib>:"Offset to CAD.vi"("Max CAD"=w42, "Cylinder TDC [Absolute CAD]"=w102, "Offset [DBTDC]"=w96) -> ("CAD [Absolute CAD]"=w114:sgl)  [unwired: 12 in]
      n77 = call <vilib>:"Offset to CAD.vi"("Max CAD"=w42, "Cylinder TDC [Absolute CAD]"=w101, "Offset [DBTDC]"=w95) -> ("CAD [Absolute CAD]"=w113:sgl)  [unwired: 12 in]
      n78 = call <vilib>:"Offset to CAD.vi"("Max CAD"=w42, "Cylinder TDC [Absolute CAD]"=w101, "Offset [DBTDC]"=w96) -> ("CAD [Absolute CAD]"=w112:sgl)  [unwired: 12 in]
      n79 = call <vilib>:"Offset to CAD.vi"("Max CAD"=w42, "Cylinder TDC [Absolute CAD]"=w104, "Offset [DBTDC]"=w70) -> ("CAD [Absolute CAD]"=w111:sgl)  [unwired: 12 in]
      n80 = call <vilib>:"Offset to CAD.vi"("Max CAD"=w42, "Cylinder TDC [Absolute CAD]"=w103, "Offset [DBTDC]"=w40) -> ("CAD [Absolute CAD]"=w110:sgl)  [unwired: 12 in]
      n81 = call <vilib>:"Offset to CAD.vi"("Max CAD"=w42, "Cylinder TDC [Absolute CAD]"=w102, "Offset [DBTDC]"=w38) -> ("CAD [Absolute CAD]"=w109:sgl)  [unwired: 12 in]
      n82 = call <vilib>:"Offset to CAD.vi"("Max CAD"=w42, "Cylinder TDC [Absolute CAD]"=w101, "Offset [DBTDC]"=w36) -> ("CAD [Absolute CAD]"=w108:sgl)  [unwired: 12 in]
      n83 = for {
        tunnel: w45 -> [w122] mode=indexing
        tunnel: [w121] -> w44 mode=indexing
        n84 = call <vilib>:"time2ticks.vi"("Time (msec)"=w122) -> ("Ticks"=w121:u32)  [unwired: 1 in]
      }
      n85 = for {
        N: 8 -> [_]
        tunnel: w69 -> [w128] mode=indexing
        tunnel: [w127] -> w54 mode=indexing
        tunnel: w44 -> [w123]
        w135 = bool[] [TRUE, FALSE, FALSE, FALSE, FALSE, FALSE, FALSE, FALSE]  # CmdLevel
        w125 = bool[] [FALSE, TRUE, TRUE, TRUE, TRUE, TRUE, TRUE, FALSE]  # Continue
        n86 = call "Hardware|ESTTL-1|Restrike1Enable"() -> ("Value"=w132:bool)
        n87 = call "Hardware|ESTTL-1|Restrike2Enable"() -> ("Value"=w133:bool)
        n88 = call "Hardware|ESTTL-1|Restrike3Enable"() -> ("Value"=w134:bool)
        n89 = Compound Arithmetic op=AND(w128, w132) -> (w131:bool)
        n90 = Compound Arithmetic op=AND(w128, w133) -> (w130:bool)
        n91 = Compound Arithmetic op=AND(w128, w134) -> (w129:bool)
        n92 = Replace Array Subset(array=w135, new element #1=w131, index #1=2 ("index"), new element #2=w130, index #2=4 ("index"), new element #3=w129, index #3=6 ("index")) -> (w126:bool[])
        n93 = Bundle By Name(cluster=T29 {"DurationSeq"=[0, 0, 0, 0, 0, 0, 0, 0, 0, 0, 0, 0, 0, 0, 0, 0], "CmdLevelSeq"=[FALSE, FALSE, FALSE, FALSE, FALSE, FALSE, FALSE, FALSE, FALSE, FALSE, FALSE, FALSE, FALSE, FALSE, FALSE, FALSE], "ContinueSeq"=[FALSE, FALSE, FALSE, FALSE, FALSE, FALSE, FALSE, FALSE, FALSE, FALSE, FALSE, FALSE, FALSE, FALSE, FALSE, FALSE]} ("Spark_Sequence"), "ContinueSeq"=w125, "CmdLevelSeq"=w126, "DurationSeq"=w123) -> (w127:T29)
      }
      n94 = call "Critical| |"() -> ("Fault"=w16:bool)  [unwired: 2 in]
      n95 = call "Hardware|ESTTL-1|DisableOnCrit"() -> ("Value"=w15:bool)
      n96 = call "Hardware|ESTTL-1|Ch1Enable"() -> ("Value"=w107:bool)
      n97 = call "Hardware|ESTTL-1|Ch2Enable"() -> ("Value"=w120:bool)
      n98 = call "Hardware|ESTTL-1|Ch3Enable"() -> ("Value"=w106:bool)
      n99 = call "Hardware|ESTTL-1|Ch4Enable"() -> ("Value"=w105:bool)
      n100 = call "Hardware|ESTTL-1|Ch5Enable"() -> ("Value"=w100:bool)
      n101 = call "Hardware|ESTTL-1|Ch6Enable"() -> ("Value"=w99:bool)
      n102 = call "Hardware|ESTTL-1|Ch7Enable"() -> ("Value"=w98:bool)
      n103 = call "Hardware|ESTTL-1|Ch8Enable"() -> ("Value"=w97:bool)
      n104 = And(x=w16, y=w15) -> (x .and. y?=w14:bool)
      n105 = Compound Arithmetic op=AND(invert w14, w107) -> (w55:bool)
      n106 = Compound Arithmetic op=AND(invert w14, w120) -> (w56:bool)
      n107 = Compound Arithmetic op=AND(invert w14, w106) -> (w57:bool)
      n108 = Compound Arithmetic op=AND(invert w14, w105) -> (w58:bool)
      n109 = Compound Arithmetic op=AND(invert w14, w100) -> (w59:bool)
      n110 = Compound Arithmetic op=AND(invert w14, w99) -> (w60:bool)
      n111 = Compound Arithmetic op=AND(invert w14, w98) -> (w61:bool)
      n112 = Compound Arithmetic op=AND(invert w14, w97) -> (w62:bool)
      n113 = xnode "Read/Write Control"("FPGA VI Reference In"=w65, "ESTTL-1.Sequences"=w54) -> ("FPGA VI Reference Out"=w64:refnum<k20>)  [unwired: 1 in, 1 out]
      n114 = Bundle By Name(cluster=T28 {"Channel Enable 1"=FALSE, "Window_Start 1 [CAD]"=0.0, "Window_End 1 [CAD]"=0.0, "Dwell 1 [ms]"=0.0, "Spark Timing 1 [CAD]"=0.0, "Channel Enable 2"=FALSE, "Window_Start 2 [CAD]"=0.0, "Window_End 2 [CAD]"=0.0, "Dwell 2 [ms]"=0.0, "Spark Timing 2 [CAD]"=0.0, "Channel Enable 3"=FALSE, "Window_Start 3 [CAD]"=0.0, "Window_End 3 [CAD]"=0.0, "Dwell 3 [ms]"=0.0, "Spark Timing 3 [CAD]"=0.0, "Channel Enable 4"=FALSE, "Window_Start 4 [CAD]"=0.0, "Window_End 4 [CAD]"=0.0, "Dwell 4 [ms]"=0.0, "Spark Timing 4 [CAD]"=0.0, "Channel Enable 5"=FALSE, "Window_Start 5 [CAD]"=0.0, "Window_End 5 [CAD]"=0.0, "Dwell 5 [ms]"=0.0, "Spark Timing 5 [CAD]"=0.0, "Channel Enable 6"=FALSE, "Window_Start 6 [CAD]"=0.0, "Window_End 6 [CAD]"=0.0, "Dwell 6 [ms]"=0.0, "Spark Timing 6 [CAD]"=0.0, "Channel Enable 7"=FALSE, "Window_Start 7 [CAD]"=0.0, "Window_End 7 [CAD]"=0.0, "Dwell 7 [ms]"=0.0, "Spark Timing 7 [CAD]"=0.0, "Channel Enable 8"=FALSE, "Window_Start 8 [CAD]"=0.0, "Window_End 8 [CAD]"=0.0, "Dwell 8 [ms]"=0.0, "Spark Timing 8 [CAD]"=0.0} ("ESTTL-1.Config"), "Channel Enable 1"=w55, "Channel Enable 2"=w56, "Channel Enable 3"=w57, "Channel Enable 4"=w58, "Channel Enable 5"=w59, "Channel Enable 6"=w60, "Channel Enable 7"=w61, "Channel Enable 8"=w62, "Window_Start 1 [CAD]"=w119, "Window_End 1 [CAD]"=w118, "Window_Start 2 [CAD]"=w117, "Window_End 2 [CAD]"=w116, "Window_Start 3 [CAD]"=w115, "Window_End 3 [CAD]"=w114, "Window_Start 4 [CAD]"=w113, "Window_End 4 [CAD]"=w112, "Dwell 1 [ms]"=w63, "Spark Timing 1 [CAD]"=w111, "Dwell 2 [ms]"=w41, "Spark Timing 2 [CAD]"=w110, "Dwell 3 [ms]"=w39, "Spark Timing 3 [CAD]"=w109, "Dwell 4 [ms]"=w37, "Spark Timing 4 [CAD]"=w108, "Window_Start 5 [CAD]"=w90, "Window_End 5 [CAD]"=w89, "Window_Start 6 [CAD]"=w88, "Window_End 6 [CAD]"=w87, "Window_Start 7 [CAD]"=w86, "Window_End 7 [CAD]"=w85, "Window_Start 8 [CAD]"=w84, "Window_End 8 [CAD]"=w83, "Dwell 5 [ms]"=w27, "Spark Timing 5 [CAD]"=w82, "Dwell 6 [ms]"=w26, "Spark Timing 6 [CAD]"=w81, "Dwell 7 [ms]"=w23, "Spark Timing 7 [CAD]"=w80, "Dwell 8 [ms]"=w21, "Spark Timing 8 [CAD]"=w79) -> (w17:T28)
      n115 = xnode "Read/Write Control"("FPGA VI Reference In"=w64, "ESTTL-1.Config"=w17) -> ()  [unwired: 1 in, 2 out]
    }
    frame Error {
    }
  }
  n116 = call "Hardware|ESTTL-1|FPGAInterfaceError"("Value"=w1) -> ()
  n117 = call "Non-Critical|ESTTL-1|FPGAInterfaceError"("Fault"=w1) -> ()  [unwired: 2 in]
